vi "Set Operating Mode.vi"(8 "error in":errorcluster, 11 "3300 in":refnum<class "3300.lvclass">) -> (0 "error out":errorcluster, 3 "3300 out":refnum<class "3300.lvclass">)   [LabVIEW 2019, in "3300.lvlib" / "3300.lvclass"]
uses:
  Library/3300.lvclass
  C:/Users/Public/Documents/Development/builds/Instruments/Electronic Load.lvlibp/Library/Electronic Load.lvclass
  Library/3300.lvclass/3300.ctl
  Accessors/Read Local Resource.vi
  Accessors/Write Local Resource.vi
  builds/Instruments/Electronic Load.lvlibp/Accessors/Settings/Read Mode.vi
  <instrlib>/Agilent N330X Series/Agilent N330X Series.lvlib
  builds/Engine/Engine.lvlibp/Project/Engine.lvclass
  C:/Users/Public/Documents/Development/builds/Engine/Engine.lvlibp/Project/Engine.lvclass
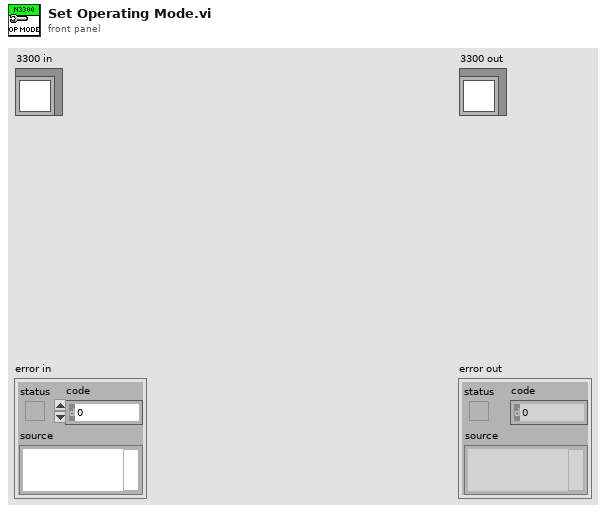
[diagram p1: front panel]
types:
  T1 = typedef "Electronic Load.lvlibp/Electronic Load.lvclass/E-Load Mode.ctl" = enum16{"Current", "Resistance", "Voltage"}
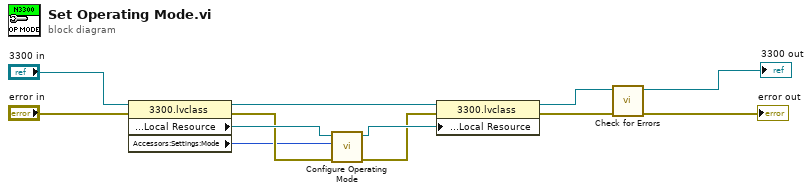
[diagram p0: block diagram]
diagram:
  n1 = property class="3300.lvclass"(reference="3300 in", error in="error in") -> (reference out=w10:refnum<class "3300.lvclass">, error out=w6:errorcluster, "Private:Accessors:Local Resource"=w9:refnum<visa-resource-name>, "Accessors:Settings:Mode"=w5:T1)
  n2 = call <instrlib>:"Configure Operating Mode.vi"("error in (no error)"=w6, "Regulation Mode (0:Current)"=w5, "VISA resource name"=w9) -> ("error out"=w7:errorcluster, "VISA resource name out"=w8:refnum<visa-resource-name>)  [unwired: 7 in]
  n3 = property class="3300.lvclass"(reference=w10, error in=w7, "Private:Accessors:Local Resource"=w8) -> (reference out=w3:refnum<class "3300.lvclass">, error out=w4:errorcluster)
  n4 = call "Check for Errors.vi"("error in"=w4, "Engine in"=w3) -> ("error out"=→"error out":errorcluster, "Engine out"=→"3300 out":refnum<class "3300.lvclass">)  [unwired: 8 in]
